vi "Type Specialization for Path.vi"(11 "error in (no error)":errorcluster) -> (4 "Type Specialization for Path":T1(array[cluster]), 15 "error out":errorcluster)   [LabVIEW 2021, in "Migrator.lvlib"]
uses:
  Migrator.lvlib
  <vilib>/Utility/traverseref.llb/TRef TravTarget.ctl
  <vilib>/Utility/traverseref.llb/VI Scripting - Traverse.lvlib
  Path Functions/Path Functions.lvlib
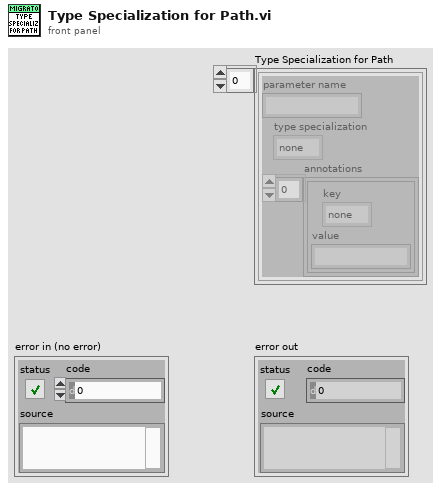
[diagram p1: front panel]
types:
  T1 = cluster{"parameter name":string, "type specialization":enum16{"none", "pin", "path", "enum"}, "annotations":cluster{"key":enum16{"none", "pin.instrument_type", "enum.values"}, "value":string}[]}[]
  T2 = typedef "TRef TravTarget.ctl" = enum16{"FP", "BD", "Other"}
  T3 = cluster{"parameter name":string, "type specialization":enum16{"none", "pin", "path", "enum"}, "annotations":cluster{"key":enum16{"none", "pin.instrument_type", "enum.values"}, "value":string}[]}
  T4 = cluster{"key":enum16{"none", "pin.instrument_type", "enum.values"}, "value":string}[]
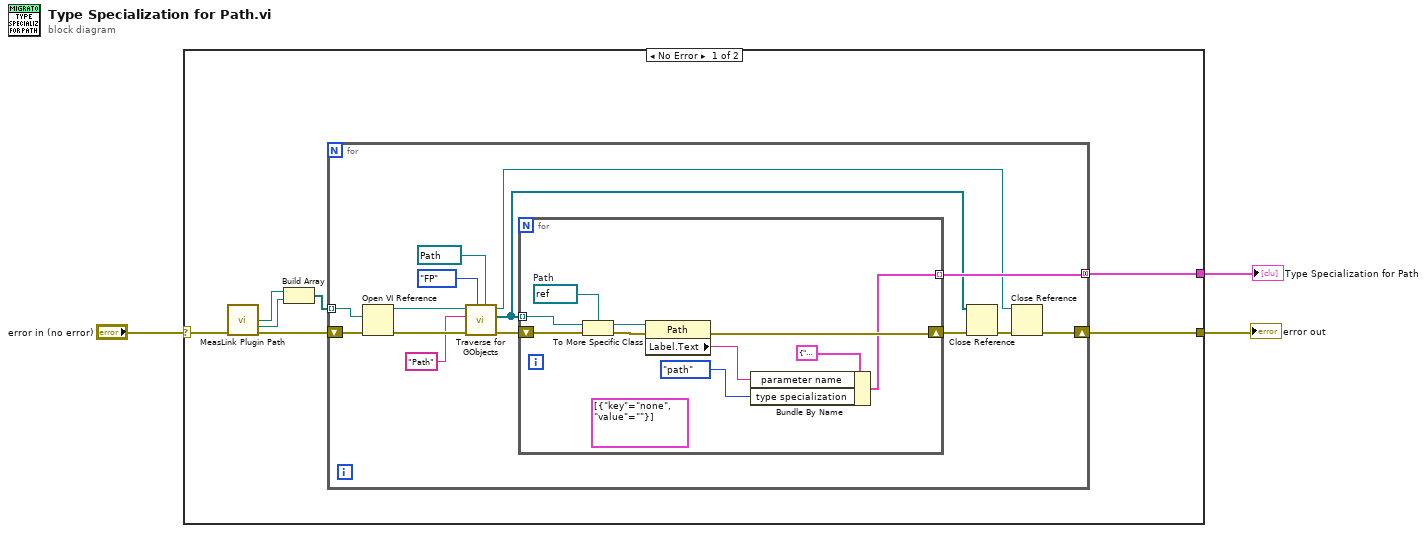
[diagram p0: block diagram]
diagram:
  n1 = case shown="No Error" "error in (no error)" {
    selector: "error in (no error)" -> [w6 w35]
    tunnel: [w5 w35] -> w2
    tunnel: [w4 _] -> w1
    frame No Error {
      n2 = call "MeasLink Plugin Path.vi"("error in (no error)"=w6) -> ("Result Control"=w10:path, "Input Controls"=w9:path, "error out"=w7:errorcluster)  [unwired: 2 in, 10 out]
      n3 = Build Array(w10, w9) -> (w8:path[])
      n4 = for {
        tunnel: w8 -> [w22] mode=indexing
        shift-right: [w12] -> w5
        shift-left: w7 -> [w23]
        tunnel: [w16] -> w4 mode=concatenating
        n5 = Open VI Reference(vi path=w22, error in (no error)=w23) -> (vi reference=w21:refnum<vi>, error out=w24:errorcluster)  [unwired: 4 in]
        n6 = call <vilib>:"Traverse for GObjects.vi"("Other Refnum"=refnum<vi> refnum, "Traverse Target"=TRef_TravTarget."FP", "error in (no error)"=w24, "Class Name"="Path", "VI Refnum"=w21) -> ("error out"=w17:errorcluster, "References"=w14:refnum<vi>[], "dup VI Refnum"=w13:refnum<vi>)  [unwired: 3 in, 1 out]
        n7 = for {
          shift-right: [w26] -> w15
          shift-left: w17 -> [w34]
          tunnel: w14 -> [w33] mode=indexing
          tunnel: [w25] -> w16 mode=indexing
          (unwired) T4 [{"key"=enum."none", "value"=""}] ("annotations")
          w32 = refnum<vi> refnum  # Path
          n8 = To More Specific Class(target class=w32, reference=w33, error in=w34) -> (specific class reference=w30:refnum<vi>, error out=w31:errorcluster)
          n9 = property class="Path"(reference=w30, error in=w31) -> (error out=w26:errorcluster, "Label.Text"=w28:string)  [unwired: 1 out]
          n10 = Bundle By Name(cluster=T3 {"parameter name"="", "type specialization"=enum."none", "annotations"=[]} ("Type Specialization"), "parameter name"=w28, "type specialization"=enum16{"none", "pin", "path", "enum"}."path") -> (w25:T3)
        }
        n11 = Close Reference(reference=w14, error in (no error)=w15) -> (error out=w11:errorcluster)
        n12 = Close Reference(reference=w13, error in (no error)=w11) -> (error out=w12:errorcluster)
      }
    }
    frame Error {
    }
  }
  "error out" <- w2
  "Type Specialization for Path" <- w1
